vi "On Start.vi"(7 "Host Resources":T1, 8 "error in (no error)":errorcluster, 11 "Hardware Configuration in":T4) -> (0 "error out":errorcluster, 3 "Hardware Configuration out":T4)   [LabVIEW 2021, in "Acquisition.lvlib"]
doc: "Initialize the data acquisition hardware references."
uses:
  Acquisition.lvlib
  Hardware Configuration.ctl
  Channel Settings.ctl
  IO Device.ctl
  Interval Timer/Repeat Interval.ctl
  Interval Timer/Interval Length.ctl
  Interval Timer/Interval Token.ctl
  IO API.ctl
  Host Resources.ctl
  Host Software Package.ctl
  Host IO Resource.ctl
  Interval Timer/Interval Timer.lvlib
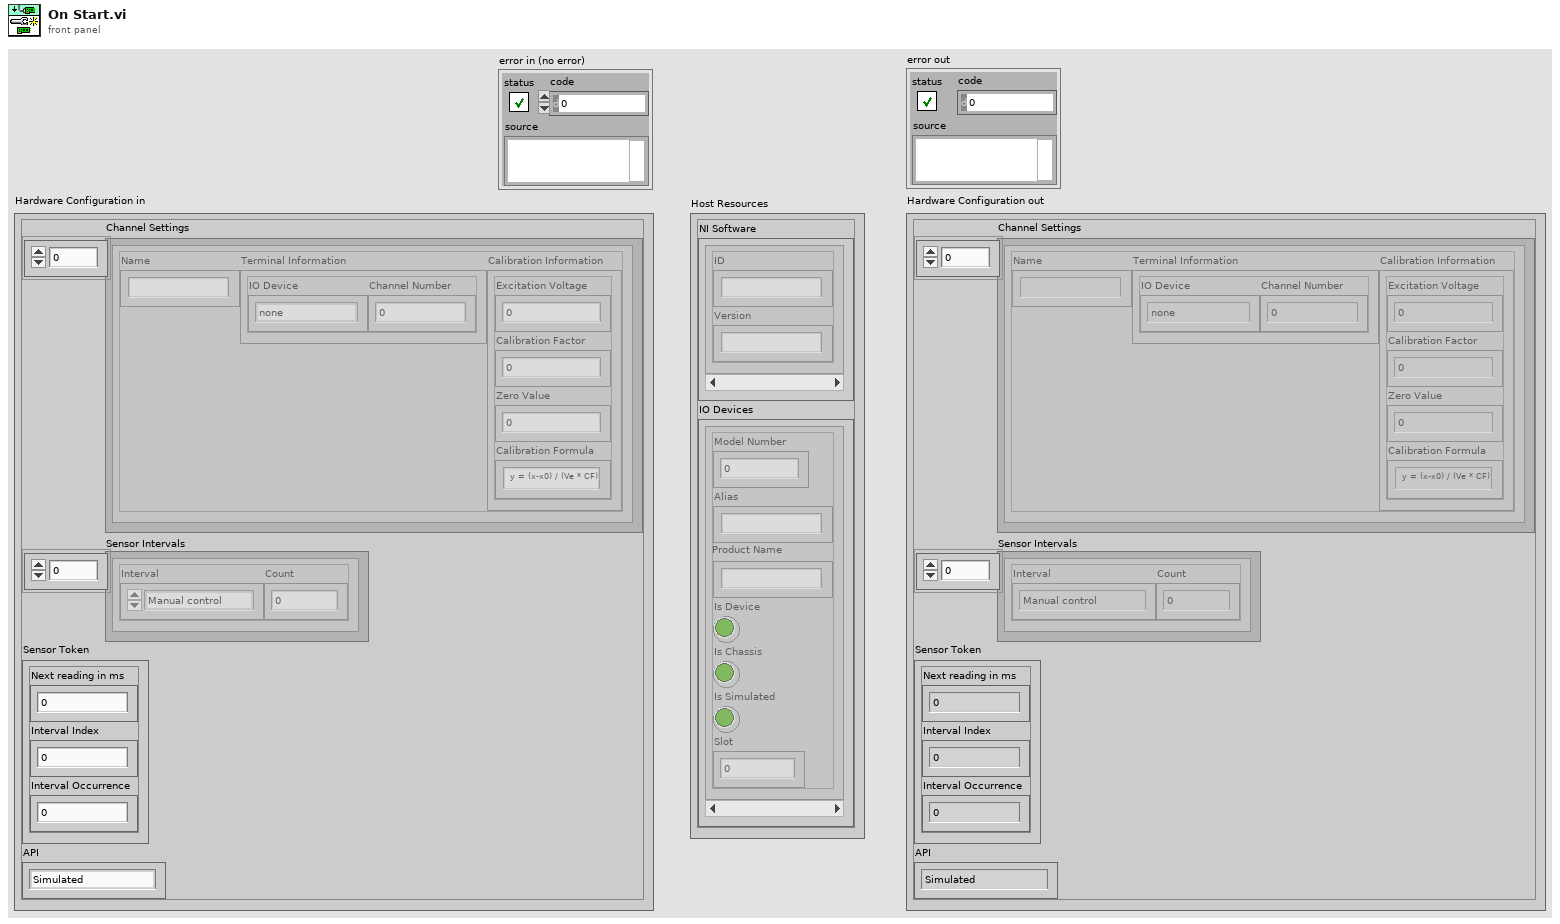
[diagram p1: front panel]
types:
  T1 = typedef "Acquisition.lvlib/Host Resources.ctl" = cluster{"NI Software":T2[], "IO Devices":T3[]}
  T2 = typedef "Acquisition.lvlib/Host Software Package.ctl" = cluster{"ID":string, "Version":string}
  T3 = typedef "Acquisition.lvlib/Host IO Resource.ctl" = cluster{"Model Number":u32, "Alias":string, "Product Name":string, "Is Device":bool, "Is Chassis":bool, "Is Simulated":bool, "Slot":i32}
  T4 = typedef "Acquisition.lvlib/Hardware Configuration.ctl" = cluster{"Channel Settings":T5[], "Sensor Intervals":T7[], "Sensor Token":T9, "API":T10}
  T5 = typedef "Acquisition.lvlib/Channel Settings.ctl" = cluster{"Name":string, "Terminal Information":cluster{"IO Device":T6, "Channel Number":i32}, "Calibration Information":cluster{"Excitation Voltage":dbl, "Calibration Factor":dbl, "Zero Value":dbl, "Calibration Formula":string}}
  T6 = typedef "Acquisition.lvlib/IO Device.ctl" = enum16{"none", "9219", "9401"}
  T7 = typedef "Interval Timer.lvlib/Repeat Interval.ctl" = cluster{"Interval":T8, "Count":i32}
  T8 = typedef "Interval Timer.lvlib/Interval Length.ctl" = enum16{"Manual control", "1 second", "10 seconds", "30 seconds", "60 seconds", "600 seconds", "1200 seconds", "3600 seconds"}
  T9 = typedef "Interval Timer.lvlib/Interval Token.ctl" = cluster{"Next reading in ms":u32, "Interval Index":i32, "Interval Occurrence":i32}
  T10 = typedef "Acquisition.lvlib/IO API.ctl" = enum16{"Simulated", "DAQmx"}
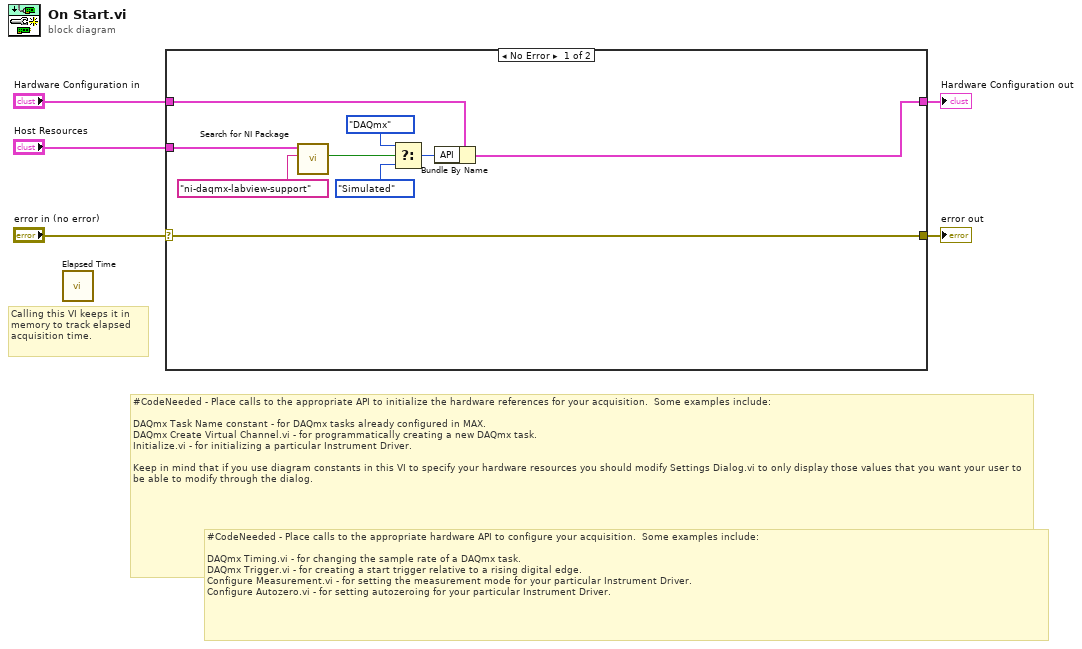
[diagram p0: block diagram]
diagram:
  # "Calling this VI keeps it in memory to track elapsed acquisition time."
  # "#CodeNeeded - Place calls to the appropriate hardware API to configure your acquisition.  Some examples include:\n\nDAQmx Timing.vi - for changing the sample rate of a DAQmx task.\nDAQmx Trigger.vi - for creating a start trigger relative to a rising digital edge.\nConfigure Measurement.vi - for setting the measurement mode for your particular Instrument Driver.\nConfigure Autozero.vi - for setting autozeroing for your particular Instrument Driver."
  # "#CodeNeeded - Place calls to the appropriate API to initialize the hardware references for your acquisition.  Some examples include:\n\nDAQmx Task Name constant - for DAQmx tasks already configured in MAX.\nDAQmx Create Virtual Channel.vi - for programmatically creating a new DAQmx task.\nInitialize.vi - for initializing a particular Instrument Driver.\n\nKeep in mind that if you use diagram constants in this VI to specify your hardware resources you should modify Settings Dialog.vi to only display those values that you want your user to be able to modify through the dialog."
  n1 = call "Elapsed Time.vi"() -> ()  [unwired: 9 in, 3 out]
  n2 = case shown="No Error" "error in (no error)" {
    selector: "error in (no error)" -> [w14 w15]
    tunnel: [w14 w15] -> w4
    tunnel: "Hardware Configuration in" -> [w8 w16]
    tunnel: [w7 w16] -> w2
    tunnel: "Host Resources" -> [w13 _]
    frame No Error {
      n3 = call "Search for NI Package.vi"("software package ID"="ni-daqmx-labview-support", "Host Resources"=w13) -> ("Is package installed?"=w11:bool)  [unwired: 9 in]
      n4 = Select(t=IO_API."DAQmx" ("API"), s=w11, f=IO_API."Simulated" ("API")) -> (s? t:f=w6:T10)
      n5 = Bundle By Name(cluster=w8, "API"=w6) -> (w7:T4)
    }
    frame Error {
    }
  }
  "Hardware Configuration out" <- w2
  "error out" <- w4
